vi "JSON Escape.vi"(8 "error in (no error)":errorcluster, 11 "String":string) -> (0 "error out":errorcluster, 2 "Characters Escaped?":bool, 3 "Escaped String":string)   [LabVIEW 2018, in "labview_json.lvlib"]
uses:
  labview_json.lvlib
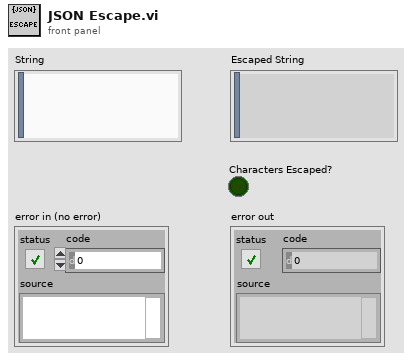
[diagram p1: front panel]
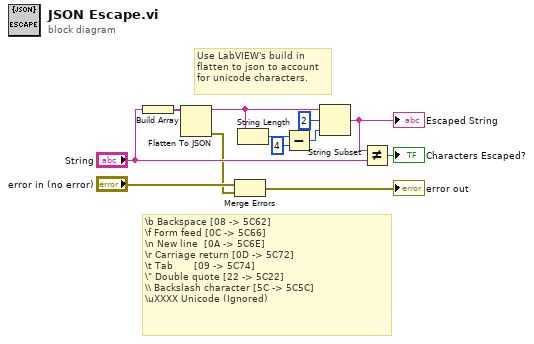
[diagram p0: block diagram]
diagram:
  # "Use LabVIEW's build in\nflatten to json to account\nfor unicode characters."
  # "\\b Backspace [08 -> 5C62]\n\\f Form feed [0C -> 5C66]\n\\n New line  [0A -> 5C6E]\n\\r Carriage return [0D -> 5C72]\n\\t Tab       [09 -> 5C74]\n\\\" Double quote [22 -> 5C22]\n\\\\ Backslash character [5C -> 5C5C]\n\\uXXXX Unicode (Ignored)"
  n1 = Build Array("String") -> (w9:string[])
  n2 = Flatten To JSON(anything=w9) -> (JSON string=w7:string, 11:w1:errorcluster)  [unwired: 2 in]
  n3 = Merge Errors("error in (no error)", w1) -> (→"error out":errorcluster)
  n4 = String Length(string=w7) -> (length=w6:i32)
  n5 = Subtract(x=w6, y=4) -> (x-y=w4:i32)
  n6 = String Subset(string=w7, offset (0)=2, length (rest)=w4) -> (substring=w12:string)
  "Escaped String" <- w12
  n7 = Not Equal?(x=w12, y="String") -> (x != y?=→"Characters Escaped?":bool)
